vi "Contains Point.vi"(8 "error in (no error)":errorcluster, 10 "point":cluster{"x":i16, "y":i16}, 11 "Port in":refnum<class "FSM.Port.lvclass">) -> (0 "error out":errorcluster, 2 "contains point":bool, 3 "Port out":refnum<class "FSM.Port.lvclass">)   [LabVIEW 2020, in "FSM.Port.lvclass"]
uses:
  FSM.Port.lvclass
  FSM.Port.lvclass/FSM.Port.ctl
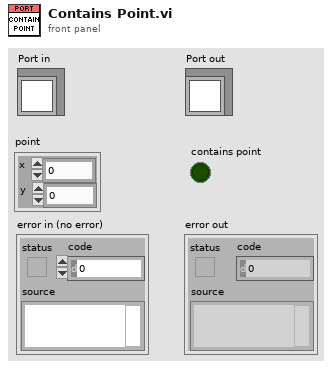
[diagram p1: front panel]
types:
  T1 = cluster{"left":i16, "top":i16, "right":i16, "bottom":i16}
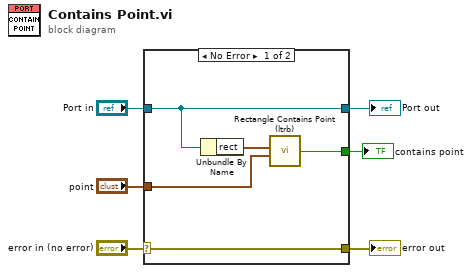
[diagram p0: block diagram]
diagram:
  n1 = case shown="No Error" "error in (no error)" {
    selector: "error in (no error)" -> [w11 w13]
    tunnel: [w11 w13] -> w5
    tunnel: [w10 w12] -> w3
    tunnel: "Port in" -> [w10 w12]
    tunnel: "point" -> [w8 _]
    tunnel: [w7 _] -> w1
    frame No Error {
      n2 = Unbundle By Name(w10) -> ("rect"=w9:T1)
      n3 = call "Rectangle Contains Point (ltrb).vi"("Point"=w8, "Rectangle"=w9) -> ("Contained?"=w7:bool)  [unwired: 4 in]
    }
    frame Error {
    }
  }
  "error out" <- w5
  "Port out" <- w3
  "contains point" <- w1
